vi "Execute Turn.vi"(7 "Player Color":T1, 8 "error in":errorcluster, 9 "Possible Moves":bool[][](array[boolean]), 10 "Board":T3[][](array[typedef]), 11 "NonOOPlayer in":refnum<class "NonOOPlayer.lvclass">) -> (0 "error out":errorcluster, 2 "Choice Coordinates":T2, 3 "NonOOPlayer out":refnum<class "NonOOPlayer.lvclass">)   [LabVIEW 2020, in "NonOOPlayer.lvclass"]
uses:
  NonOOPlayer.lvclass
  Space Ring.ctl
  Space Coordinates.ctl
  Turn Enum.ctl
  NonOOPlayer.lvclass/NonOOPlayer.ctl
  Reversi.lvclass
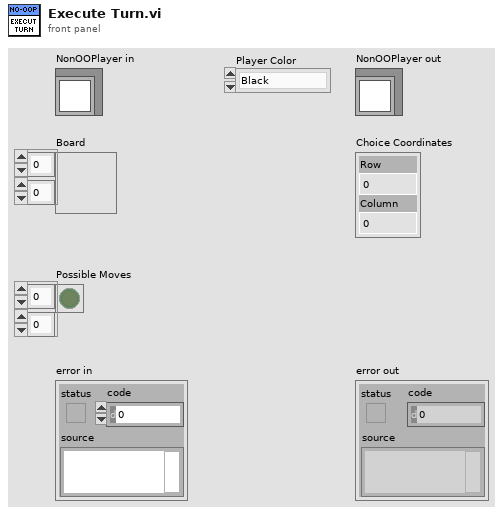
[diagram p1: front panel]
types:
  T1 = typedef "Reversi.lvlib/Reversi.lvclass/Turn Enum.ctl" = enum16{"Black", "White"}
  T2 = typedef "Reversi.lvlib/Reversi.lvclass/Space Coordinates.ctl" = cluster{"Row":i32, "Column":i32}
  T3 = typedef "Reversi.lvlib/Reversi.lvclass/Space Ring.ctl" = u16
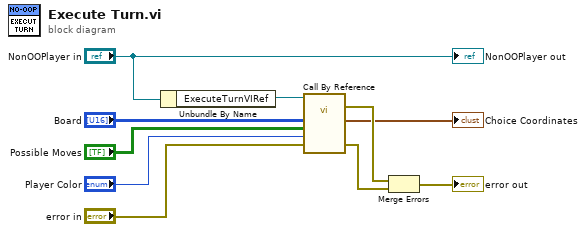
[diagram p0: block diagram]
diagram:
  n1 = Unbundle By Name("NonOOPlayer in") -> ("ExecuteTurnVIRef"=w5:refnum<vi>)
  n2 = call-by-ref "?"(reference=w5, "error in"="error in", "Player Color"="Player Color", "Possible Moves"="Possible Moves", "Board"="Board") -> (error out=w9:errorcluster, 0:"error out"=w8:errorcluster, "Choice Coordinates"=→"Choice Coordinates":T2)  [unwired: 7 in, 1 out]
  n3 = Merge Errors(w9, w8) -> (→"error out":errorcluster)
  "NonOOPlayer out" <- "NonOOPlayer in"
